vi "Get Connections per Module.vi"(8 "error in (no error)":errorcluster, 9 "Compiled Connections Indices":i32[](array[numeric]), 10 "Compiled Connection Buffer":T1[](array[typedef]), 11 "Communication Configuration":T2) -> (0 "error out":errorcluster, 3 "Connection Lists for each Module":cluster{"Indices":i32[]}[](array[cluster]))   [LabVIEW 2020, in "Routing and Faulting Engine.lvlib"]
uses:
  Routing and Faulting Engine.lvlib
  Shared/Communication Configuration.ctl
  Shared/Compiled Connection.ctl
  Shared/Routing and Faulting Shared.lvlib
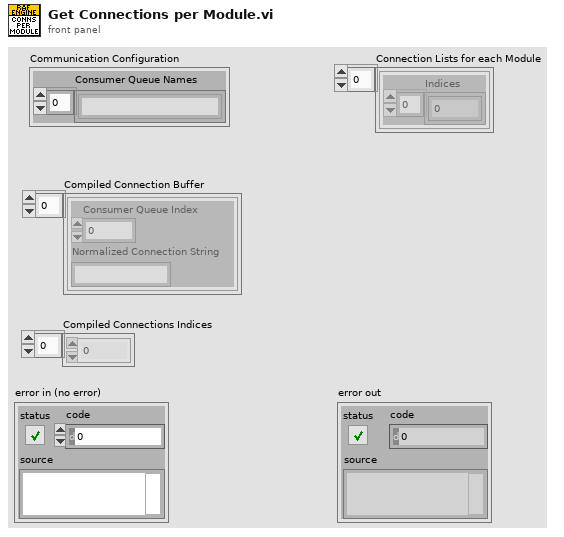
[diagram p1: front panel]
types:
  T1 = typedef "Routing and Faulting Shared.lvlib/Compiled Connection.ctl" = cluster{"Consumer Queue Index":i32, "Normalized Connection String":string}
  T2 = typedef "Routing and Faulting Shared.lvlib/Communication Configuration.ctl" = cluster{"Consumer Queue Names":string[]}
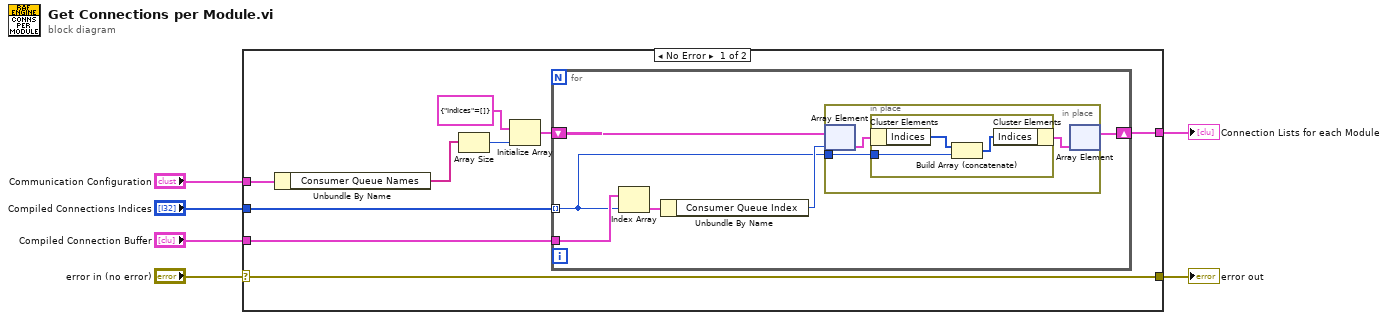
[diagram p0: block diagram]
diagram:
  n1 = case shown="No Error" "error in (no error)" {
    selector: "error in (no error)" -> [w10 w28]
    tunnel: "Compiled Connections Indices" -> [w15 _]
    tunnel: [w13 _] -> w1
    tunnel: "Communication Configuration" -> [w11 _]
    tunnel: [w10 w28] -> w4
    tunnel: "Compiled Connection Buffer" -> [w8 _]
    frame No Error {
      n2 = Unbundle By Name(w11) -> ("Consumer Queue Names"=w9:string[])
      n3 = Array Size(array=w9) -> (size(s)=w12:i32)
      n4 = Initialize Array(cluster{"Indices":i32[]} {"Indices"=[]}, w12) -> (w14:cluster{"Indices":i32[]}[])
      n5 = for {
        tunnel: w15 -> [w16] mode=indexing
        shift-right: [w20] -> w13
        shift-left: w14 -> [w21]
        tunnel: w8 -> [w19]
        n6 = Index Array(array=w19, index=w16) -> (element=w18:T1)
        n7 = Unbundle By Name(w18) -> ("Consumer Queue Index"=w17:i32)
        n8 = in-place {
          in-place-border: w16 -> [w24]
          n9 = in-place-array #1(w21, w17) -> (w23:cluster{"Indices":i32[]})
          n10 = in-place {
            in-place-border: w24 -> [w27]
            n11 = in-place-cluster #2(w23) -> ("Indices"=w26:i32[])
            n12 = Build Array (concatenate)(w26, w27) -> (w25:i32[])
            n13 = in-place-cluster #2("Indices"=w25) -> (w22:cluster{"Indices":i32[]})
          }
          n14 = in-place-array #1(w22) -> (w20:cluster{"Indices":i32[]}[])  [unwired: 1 out]
        }
      }
    }
    frame Error {
    }
  }
  "error out" <- w4
  "Connection Lists for each Module" <- w1
